vi "compound-numbers.vi"() -> ()   [LabVIEW 2025]
panel:
  out "result":dbl
  in  "Numeric 3":dbl
  in  "Numeric 2":dbl
  in  "Numeric":dbl
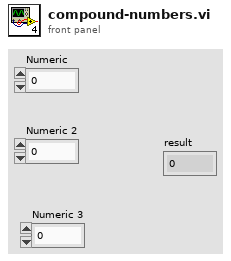
[diagram p1: front panel]
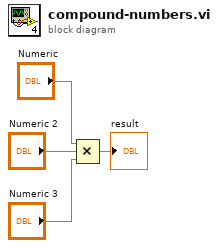
[diagram p0: block diagram]
diagram:
  n1 = Compound Arithmetic op=MULTIPLY("Numeric", "Numeric 2", "Numeric 3") -> (→"result":dbl)
